vi "THERM0dll.vi"(8 "error in (no error)":errorcluster, 9 "z":dbl[](array[numeric]), 10 "d":dbl, 11 "t":dbl) -> (0 "error out":errorcluster, 3 "Outputs":T1)   [LabVIEW 2016]
doc: "subroutine THERM0dll(t, d, z, p, e, h, s, cv, cp, w, a, g)\n\nCompute ideal-gas thermal quantities as a function of temperature, density, and composition from core functions.\nThis routine is the same as THERM, except it only calculates ideal gas properties (Z=1) at any temperature and\ndensity.\n\nINPUTS:\nt -- Temperature [K]\nd -- Molar density [mol/L]\nz -- Composition (array of mole fractions)\n\nOUTPUTS:\np -- pressure [kPa]\ne -- internal energy [J/mol]\nh -- enthalpy [J/mol]\ns -- entropy [J/mol-K]\ncv -- isochoric heat capacity [J/mol-K]\ncp -- isobaric heat capacity [J/mol-K]\nw -- speed of sound [m/s]\na -- Helmholtz energy [J/mol]\ng -- Gibbs free energy [J/mol]"
uses:
  REFPROP.DLL
panel:
  # "REFPROP-THERM0dll.vi"
  # "void  THERM0dll(double *t, double *d, double *z, double *p, double *e, double *h, double *s, double *cv, double *cp, double *w, double *a, double *g);"
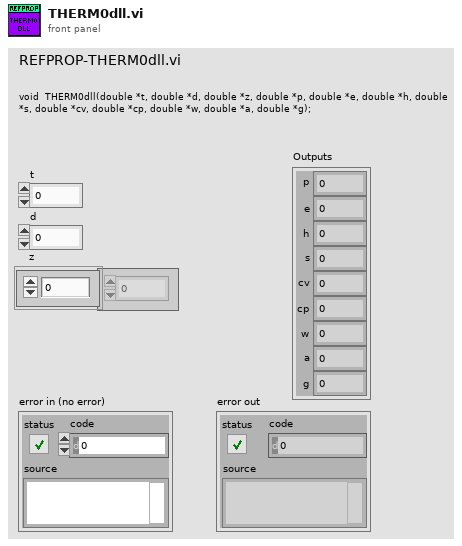
[diagram p1: front panel]
types:
  T1 = cluster{"p":dbl, "e":dbl, "h":dbl, "s":dbl, "cv":dbl, "cp":dbl, "w":dbl, "a":dbl, "g":dbl}
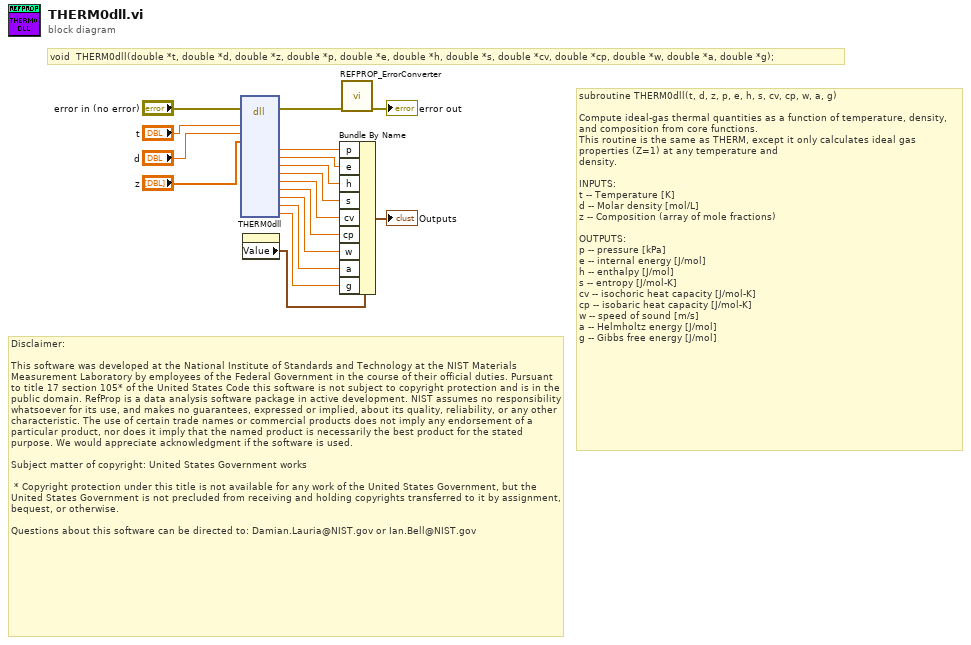
[diagram p0: block diagram]
diagram:
  # "Disclaimer:\n\nThis software was developed at the National Institute of Standards and Technology at the NIST Materials Measurement Laboratory by employees of the Federal Government in the course of their official duties. Pursuant to title 17 section 105* of the United States Code this software is not subject to copyright protection and is in the public domain. RefProp is a data analysis software package in active development. NIST assumes no responsibility whatsoever for its use, and makes no guarantees, expressed or implied, about its quality, reliability, or any other characteristic. The use of certain trade names or commercial products does not imply any endorsement of a particular product, nor does it imply that the named product is necessarily the best product for the stated purpose. We would appreciate acknowledgment if the software is used.\n \nSubject matter of copyright: United States Government works\n  \n * Copyright protection under this title is not available for any work of the United States Government, but the United States Government is not precluded from receiving and holding copyrights transferred to it by assignment, bequest, or otherwise.\n\nQuestions about this software can be directed to: Damian.Lauria@NIST.gov or Ian.Bell@NIST.gov"
  # "void  THERM0dll(double *t, double *d, double *z, double *p, double *e, double *h, double *s, double *cv, double *cp, double *w, double *a, double *g);"
  # "subroutine THERM0dll(t, d, z, p, e, h, s, cv, cp, w, a, g)\n\nCompute ideal-gas thermal quantities as a function of temperature, density, and composition from core functions.\nThis routine is the same as THERM, except it only calculates ideal gas properties (Z=1) at any temperature and\ndensity.\n\nINPUTS:\nt -- Temperature [K]\nd -- Molar density [mol/L]\nz -- Composition (array of mole fractions)\n\nOUTPUTS:\np -- pressure [kPa]\ne -- internal energy [J/mol]\nh -- enthalpy [J/mol]\ns -- entropy [J/mol-K]\ncv -- isochoric heat capacity [J/mol-K]\ncp -- isobaric heat capacity [J/mol-K]\nw -- speed of sound [m/s]\na -- Helmholtz energy [J/mol]\ng -- Gibbs free energy [J/mol]"
  n1 = dll-call lib="S:/009 - Testing/02 - Performance Testing/REFPROP/REFPROP.*" fn="THERM0dll"(error in="error in (no error)", "t"="t", "d"="d", "z"="z") -> (error out=w17:errorcluster, "p"=w1:dbl, "e"=w2:dbl, "h"=w3:dbl, "s"=w4:dbl, "cv"=w5:dbl, "cp"=w6:dbl, "w"=w7:dbl, "a"=w8:dbl, "g"=w9:dbl)  [unwired: 15 in, 1 out]
  n2 = property on="Outputs" class="Clust (strict)"() -> ("Value"=w11:T1)  [unwired: 2 in, 2 out]
  n3 = Bundle By Name(cluster=w11, "p"=w1, "e"=w2, "h"=w3, "s"=w4, "cv"=w5, "cp"=w6, "w"=w7, "a"=w8, "g"=w9) -> (→"Outputs":T1)
  n4 = call "REFPROP_ErrorConverter.vi"("error in (no error)"=w17) -> ("error out"=→"error out":errorcluster)  [unwired: 10 in]
